vi "파워 시리얼.vi"() -> ()   [LabVIEW 2018]
uses:
  <vilib>/Instr/_visa.llb/VISA Configure Serial Port (Instr).vi
panel:
  out "에러 출력":errorcluster
  in  "정지":bool
  out "버퍼 읽기":string
  out "visa":T1
  in  "문자열":string
  in  "확인 버튼":bool
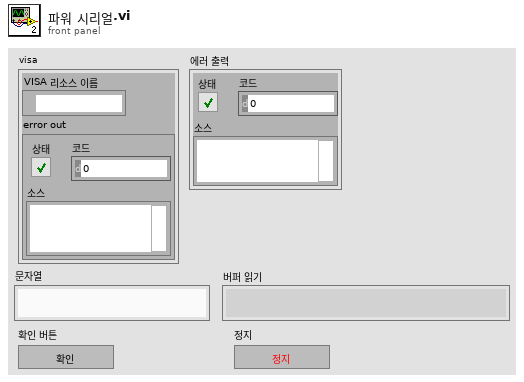
[diagram p1: front panel]
types:
  T1 = cluster{"VISA 리소스 이름":refnum<visa-resource-name>, "error out":errorcluster}
  T2 = cluster{"VISA resource name out":refnum<visa-resource-name>, "error out":errorcluster}
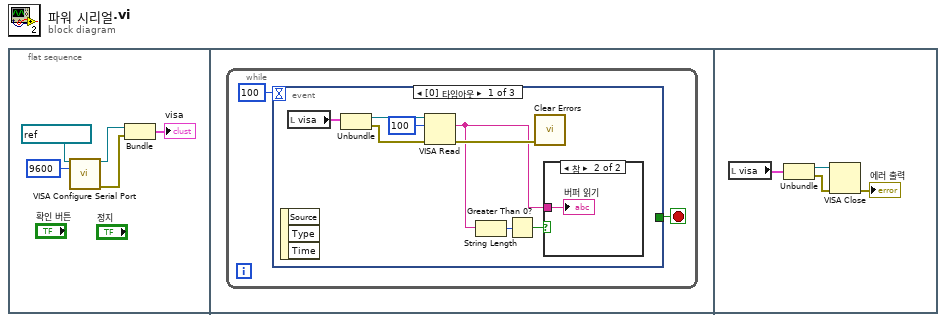
[diagram p0: block diagram]
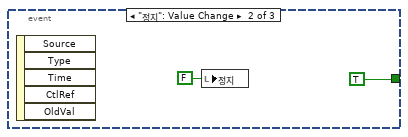
[diagram p3: hidden frame]
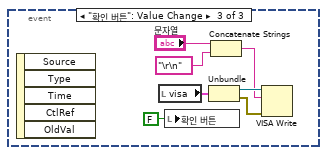
[diagram p4: hidden frame]
diagram:
  n1 = flat-sequence {
    frame #0 {
      n2 = call-poly "VISA Configure Serial Port"("VISA resource name"=refnum<visa-resource-name> "COM23", "baud rate (9600)"=u32 9600) -> ("VISA resource name out"=w4:refnum<visa-resource-name>, "error out"=w3:errorcluster)  [unwired: 12 in]
      n3 = Bundle("VISA resource name out"=w4, "error out"=w3) -> (→"visa":T2)  [unwired: 1 in]
    }
    frame #1 {
      n4 = while {
        stop <- w6 stop-if-true
        n5 = event shown="[0] 타임아웃" {
          selector: _ -> [_ _ _]
          dyn-events: _ -> [_ _ _]
          timeout: 100 -> [_ _ _]
          tunnel: [_ TRUE _] -> w6
          event Timeout {
            n6 = event-data() -> ()  [unwired: 1 in, 3 out]
            n7 = local read "visa"() -> (w15:T1)
            n8 = Unbundle(w15) -> ("VISA 리소스 이름"=w14:refnum<visa-resource-name>, "error out"=w13:errorcluster)
            n9 = VISA Read(VISA resource name=w14, byte count=u32 100 ("바이트 카운트"), error in (no error)=w13) -> (read buffer=w10:string, error out=w11:errorcluster)  [unwired: 2 out]
            n10 = String Length(string=w10) -> (length=w9:i32)
            n11 = Greater Than 0?(x=w9) -> (x > 0?=w8:bool)
            n12 = call <vilib>:"Clear Errors.vi"("error in (no error)"=w11) -> ()  [unwired: 5 in, 2 out]
            n13 = case shown="참" w8 {
              tunnel: w10 -> [_ w16]
              frame False {
              }
              frame True {
                "버퍼 읽기" <- w16
              }
            }
          }
          event "정지": Value Change {
            n14 = event-data() -> ()  [unwired: 1 in, 5 out]
            n15 = local write "정지"(FALSE ("정지")) -> ()
          }
          event "확인 버튼": Value Change {
            n16 = event-data() -> ()  [unwired: 1 in, 5 out]
            n17 = local read "visa"() -> (w24:T1)
            n18 = local write "확인 버튼"(FALSE ("확인 버튼")) -> ()
            n19 = Unbundle(w24) -> ("VISA 리소스 이름"=w23:refnum<visa-resource-name>, "error out"=w22:errorcluster)
            n20 = Concatenate Strings("문자열", "\r\n" ("문자열")) -> (w20:string)
            n21 = VISA Write(VISA resource name=w23, write buffer=w20, error in (no error)=w22) -> ()  [unwired: 3 out]
          }
        }
      }
    }
    frame #2 {
      n22 = local read "visa"() -> (w29:T1)
      n23 = Unbundle(w29) -> ("VISA 리소스 이름"=w28:refnum<visa-resource-name>, "error out"=w27:errorcluster)
      n24 = VISA Close(VISA resource name=w28, error in (no error)=w27) -> (error out=→"에러 출력":errorcluster)
    }
  }
